vi "Check Action.vi"(8 "error in (no error)":errorcluster, 10 "Action":string, 11 "Session in":refnum<class "Session.lvclass">) -> (0 "error out":errorcluster, 2 "Allowed?":bool, 3 "Session out":refnum<class "Session.lvclass">)   [LabVIEW 2016, in "Session.lvclass"]
uses:
  Session.lvclass
  Session.lvclass/Session.ctl
  Policies/Policies.lvclass
  Credentials/Credentials.lvclass
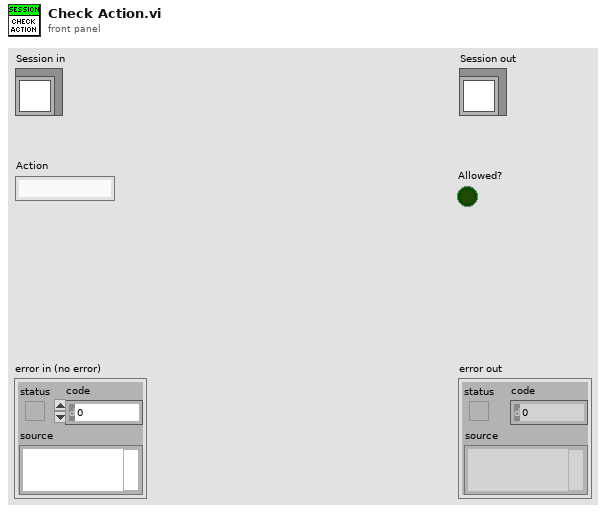
[diagram p1: front panel]
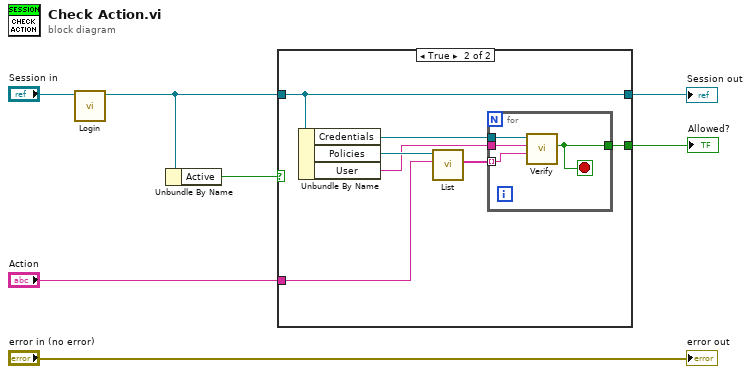
[diagram p0: block diagram]
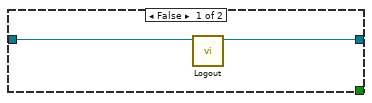
[diagram p2: hidden frame]
diagram:
  n1 = call "Login.vi"("Session in"="Session in") -> ("Session out"=w2:refnum<class "Session.lvclass">)  [unwired: 9 in, 1 out]
  n2 = Unbundle By Name(w2) -> ("Active"=w1:bool)
  n3 = case shown="True" w1 {
    tunnel: w2 -> [w9 w11]
    tunnel: "Action" -> [_ w15]
    tunnel: [_ w12] -> w4
    tunnel: [w8 w11] -> w3
    frame False {
      n4 = call "Logout.vi"("Session in"=w9) -> ("Session out"=w8:refnum<class "Session.lvclass">)  [unwired: 9 in, 1 out]
    }
    frame True {
      n5 = Unbundle By Name(w11) -> ("Credentials"=w14:refnum<class "Credentials.lvclass">, "Policies"=w16:refnum<class "Policies.lvclass">, "User"=w10:string)
      n6 = call "List.vi"("Action"=w15, "Policies in"=w16) -> ("Roles"=w13:string[])  [unwired: 7 in, 2 out]
      n7 = for {
        tunnel: w14 -> [w20]
        tunnel: w10 -> [w19]
        tunnel: w13 -> [w18] mode=indexing
        tunnel: [w17] -> w12
        stop <- w17 stop-if-true
        n8 = call "Verify.vi"("Role"=w18, "User"=w19, "Credentials in"=w20) -> ("Verified?"=w17:bool)  [unwired: 6 in, 2 out]
      }
    }
  }
  "Session out" <- w3
  "Allowed?" <- w4
  "error out" <- "error in (no error)"
